vi "READ_ACT_ENC.vi"() -> (1 "R ACT POS":fxp<+,53,21>, 2 "L ACT POS":fxp<+,53,21>)   [LabVIEW 2019]
uses:
  <vilib>/Platform/TimedLoop/XDataNode/timing_clust.ctl
  <vilib>/Platform/TimedLoop/XDataNode/nitl_modes.ctl
  <vilib>/Platform/TimedLoop/XDataNode/wakeup.ctl
  <vilib>/rvi/Emulation/niFpgaSctlEmulationGetInTimedLoop.vi
  <vilib>/rvi/Emulation/niFpgaEmulationReportErrorSimple.vi
  <vilib>/rvi/Emulation/niFpgaGetClockAttributes.vi
  <vilib>/rvi/Emulation/niFpgaCriticalErrorInLSC.vi
  <vilib>/rvi/eio/common/nirviEmuTemplateMethod_errors.vi
  <vilib>/platform/TimedLoop/XDataNode/XDataNode.xnode
  <vilib>/eio/EIONode/EIONode.xnode
  <vilib>/Platform/TimedLoop/XDataNode/XDNodeRunTimeDep.lvlib
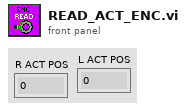
[diagram p1: front panel]
types:
  T1 = typedef "XDNodeRunTimeDep.lvlib/timing_clust.ctl" = cluster{"Expected End [f-1]":u64, "Actual End [f-1]":u64, "Finished Late? [f-1]":bool, "Expected End [i-1]":u64, "Actual End [i-1]":u64, "Finished Late? [i-1]":bool, "Expected Start [i]":u64, "Actual Start [i]":u64, "Expected Start [f]":u64, "Actual Start [f]":u64, "Source Name":string, "Structure Name":string, "Period":i64, "Deadline":i64, "Offset":i64, "Start":i64, "Priority":i32, "Timeout":i32, "Mode":T2, "Wakeup Reason":T3, "Error":errorcluster, "Source Type":string, "Secondary Source Type":string, "Global End Time":u64, "Global Start Time":u64, "Frame Duration":u64, "Iteration Duration":u64, "Assigned CPU":i32, "I/O Scan Engine Mode":u32}
  T2 = typedef "XDNodeRunTimeDep.lvlib/nitl_modes.ctl" = enum32{"No Change", "Process missed periods, maintain original phase", "Discard missed periods, maintain original phase", "Process missed periods, ignore original phase", "Discard missed periods, ignore original phase"}
  T3 = typedef "XDNodeRunTimeDep.lvlib/wakeup.ctl" = enum32{"Normal", "Aborted", "Asynchronous wakeup", "Timing source error", "Timed loop error", "Timeout"}
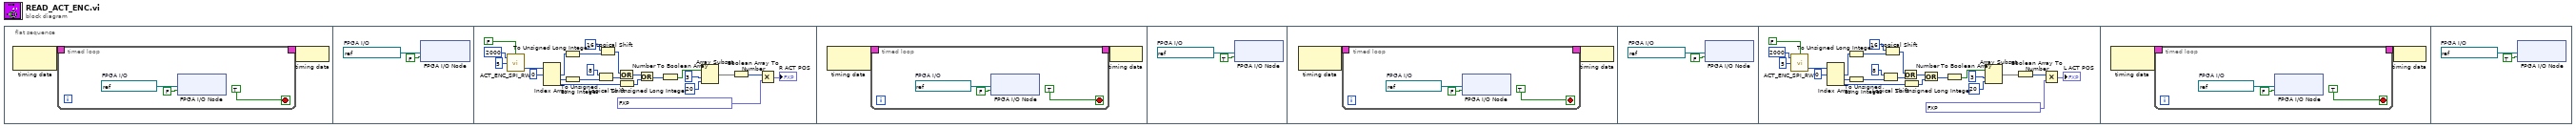
[diagram p0: block diagram]
diagram:
  n1 = flat-sequence {
    frame #0 {
      n2 = node-c288() -> (w2:T1)  [unwired: 1 in]
      n3 = timed-loop {
        timing: w2 -> [_]
        timing-out: [_] -> w1
        stop <- TRUE stop-if-true
        w4 = refnum<k21> "ACT ENC CLK"  # FPGA I/O
        n4 = xnode "FPGA I/O Node"("I/O Item"=FALSE, "FPGA I/O In"=w4) -> ()  [unwired: 1 out]
      }
      n5 = node-c288(w1) -> ()
    }
    frame #1 {
      w11 = refnum<k21> "R ACT ENC CS"  # FPGA I/O
      n6 = xnode "FPGA I/O Node"("I/O Item"=FALSE, "FPGA I/O In"=w11) -> ()  [unwired: 1 out]
    }
    frame #2 {
      n7 = call "ACT_ENC_SPI_RW.vi"("CPOL"=FALSE, "Frames to Write"=u8 5, "SPI Frequency (KHz)"=u16 2000) -> ("Data Read"=w32:u8[])  [unwired: 1 in, 1 out]
      n8 = Index Array(array=w32, index #1=0 ("index")) -> (element #1=w31:u8, element #2=w30:u8, element #3=w29:u8)  [unwired: 2 in]
      n9 = To Unsigned Long Integer(number=w31) -> (unsigned 32bit integer=w27:u32)
      n10 = To Unsigned Long Integer(number=w30) -> (unsigned 32bit integer=w25:u32)
      n11 = Logical Shift(y=i16 8, x=w25) -> (x << y=w23:u32)
      n12 = Logical Shift(y=i16 16, x=w27) -> (x << y=w24:u32)
      n13 = Or(x=w24, y=w23) -> (x .or. y?=w22:u32)
      n14 = To Unsigned Long Integer(number=w29) -> (unsigned 32bit integer=w21:u32)
      n15 = Or(x=w22, y=w21) -> (x .or. y?=w20:u32)
      n16 = Number To Boolean Array(number=w20) -> (Boolean array=w19:bool[])
      n17 = Array Subset(array=w19, index=3, length=20) -> (w16:bool[])
      n18 = Boolean Array To Number(Boolean array=w16) -> (number=w15:u32)
      n19 = Multiply(x=w15, y=fxp<+,21,-11> 0.00034332298673689365) -> (x*y=→"R ACT POS":fxp<+,53,21>)
    }
    frame #3 {
      n20 = node-c288() -> (w37:T1)  [unwired: 1 in]
      n21 = timed-loop {
        timing: w37 -> [_]
        timing-out: [_] -> w36
        stop <- TRUE stop-if-true
        w39 = refnum<k21> "ACT ENC CLK"  # FPGA I/O
        n22 = xnode "FPGA I/O Node"("I/O Item"=FALSE, "FPGA I/O In"=w39) -> ()  [unwired: 1 out]
      }
      n23 = node-c288(w36) -> ()
    }
    frame #4 {
      w46 = refnum<k21> "R ACT ENC CS"  # FPGA I/O
      n24 = xnode "FPGA I/O Node"("I/O Item"=TRUE, "FPGA I/O In"=w46) -> ()  [unwired: 1 out]
    }
    frame #5 {
      n25 = node-c288() -> (w48:T1)  [unwired: 1 in]
      n26 = timed-loop {
        timing: w48 -> [_]
        timing-out: [_] -> w47
        stop <- TRUE stop-if-true
        w50 = refnum<k21> "ACT ENC CLK"  # FPGA I/O
        n27 = xnode "FPGA I/O Node"("I/O Item"=FALSE, "FPGA I/O In"=w50) -> ()  [unwired: 1 out]
      }
      n28 = node-c288(w47) -> ()
    }
    frame #6 {
      w57 = refnum<k21> "L ACT ENC CS"  # FPGA I/O
      n29 = xnode "FPGA I/O Node"("I/O Item"=FALSE, "FPGA I/O In"=w57) -> ()  [unwired: 1 out]
    }
    frame #7 {
      n30 = call "ACT_ENC_SPI_RW.vi"("CPOL"=FALSE, "Frames to Write"=u8 5, "SPI Frequency (KHz)"=u16 2000) -> ("Data Read"=w59:u8[])  [unwired: 1 in, 1 out]
      n31 = Index Array(array=w59, index #1=0 ("index")) -> (element #1=w78:u8, element #2=w77:u8, element #3=w76:u8)  [unwired: 2 in]
      n32 = To Unsigned Long Integer(number=w78) -> (unsigned 32bit integer=w74:u32)
      n33 = To Unsigned Long Integer(number=w77) -> (unsigned 32bit integer=w72:u32)
      n34 = Logical Shift(y=i16 8, x=w72) -> (x << y=w70:u32)
      n35 = Logical Shift(y=i16 16, x=w74) -> (x << y=w71:u32)
      n36 = Or(x=w71, y=w70) -> (x .or. y?=w69:u32)
      n37 = To Unsigned Long Integer(number=w76) -> (unsigned 32bit integer=w68:u32)
      n38 = Or(x=w69, y=w68) -> (x .or. y?=w67:u32)
      n39 = Number To Boolean Array(number=w67) -> (Boolean array=w66:bool[])
      n40 = Array Subset(array=w66, index=3, length=20) -> (w63:bool[])
      n41 = Boolean Array To Number(Boolean array=w63) -> (number=w62:u32)
      n42 = Multiply(x=w62, y=fxp<+,21,-11> 0.00034332298673689365) -> (x*y=→"L ACT POS":fxp<+,53,21>)
    }
    frame #8 {
      n43 = node-c288() -> (w83:T1)  [unwired: 1 in]
      n44 = timed-loop {
        timing: w83 -> [_]
        timing-out: [_] -> w82
        stop <- TRUE stop-if-true
        w85 = refnum<k21> "ACT ENC CLK"  # FPGA I/O
        n45 = xnode "FPGA I/O Node"("I/O Item"=FALSE, "FPGA I/O In"=w85) -> ()  [unwired: 1 out]
      }
      n46 = node-c288(w82) -> ()
    }
    frame #9 {
      w92 = refnum<k21> "L ACT ENC CS"  # FPGA I/O
      n47 = xnode "FPGA I/O Node"("I/O Item"=TRUE, "FPGA I/O In"=w92) -> ()  [unwired: 1 out]
    }
  }
